vi "ReadSetpoint.vi"(11 "Device Data in":T1 {"IDS" format="%.0x"; "IDL" format="%.0x"; "IDM" format="%.0x"; "IDH" format="%.0x"}) -> (0 "Error Out":errorcluster, 1 "SetPoint %":sgl, 2 "Device Data out":T1 {"IDS" format="%.0x"; "IDL" format="%.0x"; "IDM" format="%.0x"; "IDH" format="%.0x"}, 3 "Function Output Comment":string, 4 "Unit":string, 5 "Message":string, 6 "SetPointValue":sgl)   [LabVIEW 2019]
uses:
  Device Data.ctl
  164J027_AD/Brooks DLL 1.0.1.0 32bit/Brooks DLL 1.0.1.0 Release 10032016/S Protocol/BrooksDLL.dll
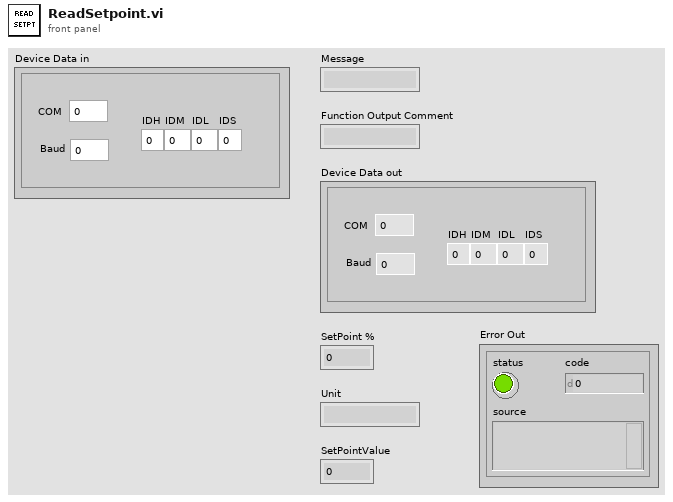
[diagram p1: front panel]
types:
  T1 = typedef "Device Data.ctl" = cluster{"COM":i32, "Baud":i32, "IDH":u8, "IDM":u8, "IDL":u8, "IDS":u8}
  T2 = cluster{bool, i32, "Function Output Comment":string}
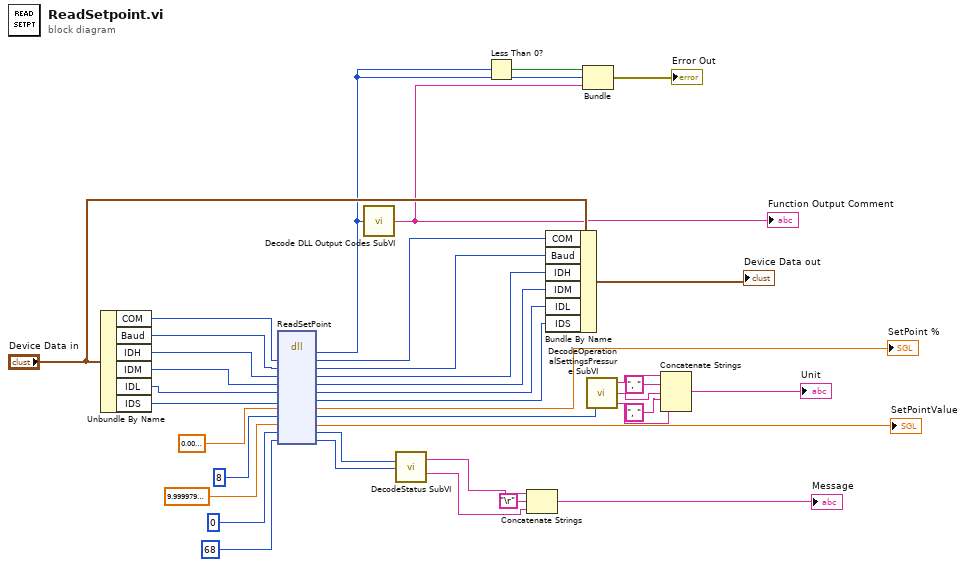
[diagram p0: block diagram]
diagram:
  n1 = Unbundle By Name("Device Data in") -> ("COM"=w23:i32, "Baud"=w24:i32, "IDH"=w28:u8, "IDM"=w27:u8, "IDL"=w26:u8, "IDS"=w25:u8)
  n2 = dll-call lib="G:/Developpement_de_Programmes/Programmes/Controle de pression/164J027_AD/Brooks DLL 1.0.1.0 32bit/Brooks DLL 1.0.1.0 Release 10032016/S Protocol/BrooksDLL.dll" fn="ReadSetPoint"("COM"=w23, "Baud"=w24, "IDH"=w28, "IDM"=w27, "IDL"=w26, "IDS"=w25, "SetPoint"=sgl 0.01 ("SetPoint %"), "FlowUnit"=u8 8 ("Unit Code"), "SetPointValue"=sgl 9.999979 ("Set Point Value"), "S1"=u8 0, "S2"=u8 68) -> (w3:i32, "COM"=w34:i32, "Baud"=w35:i32, "IDH"=w33:u8, "IDM"=w32:u8, "IDL"=w31:u8, "IDS"=w30:u8, "SetPoint"=→"SetPoint %":sgl, "FlowUnit"=w7:u8, "SetPointValue"=→"SetPointValue":sgl, "S1"=w6:u8, "S2"=w5:u8)  [unwired: 3 in, 2 out]
  n3 = call "Decode DLL Output Codes SubVI.vi"("Numeric"=w3) -> ("Function Output Comment"=w2:string)
  "Function Output Comment" <- w2
  n4 = call "DecodeStatus SubVI.vi"("S2"=w5, "S1"=w6) -> ("S2 String"=w10:string, "S1 String"=w9:string)
  n5 = Less Than 0?(x=w3) -> (x < 0?=w4:bool)
  n6 = Concatenate Strings(w9, "\r" ("string"), w10) -> (→"Message":string)
  n7 = Bundle By Name(cluster="Device Data in", "COM"=w34, "Baud"=w35, "IDH"=w33, "IDM"=w32, "IDL"=w31, "IDS"=w30) -> (→"Device Data out":T1)
  n8 = Bundle(w4, w3, "Function Output Comment"=w2) -> (→"Error Out":T2)  [unwired: 1 in]
  n9 = call "DecodeOperationalSettingsPressure SubVI.vi"("PressureUnitCode"=w7) -> ("PressureMode Comment"=w16:string, "Pressure Reference Comment"=w14:string, "PressureUnitCode Comment"=w12:string)  [unwired: 2 in]
  n10 = Concatenate Strings(w12, ", ", w14, ", ", w16) -> (→"Unit":string)
